vi "LV6_3.vi"() -> ()   [LabVIEW 2016]
uses:
  <vilib>/sound2/lvsound2.llb/Sampling Mode.ctl
  <vilib>/Utility/file.llb/Read From Spreadsheet File (DBL).vi
  <vilib>/imath/engines/lvmath2/RunTimeEngine/BuiltInFunctions/length/NIMS_length(GV).vi
  <instcachedir>/0/NIMS_length(GV)_08A3D13377FD4E4B96F5795FBF3698FA.lvgen/NIMS_length(GV)_08A3D13377FD4E4B96F5795FBF3698FA_000.vi
  <vilib>/imath/engines/lvmath2/RunTimeEngine/RangeToken/NIMS_Range.vi
  <instcachedir>/0/NIMS_Range_A7C094595B484CA7AF10685B02D808ED.lvgen/NIMS_Range_A7C094595B484CA7AF10685B02D808ED_001.vi
  <vilib>/imathl/engines/lvmath/Functions/Error Handling/Create Error.vi
  <vilib>/imath/engines/lvmath2/RunTimeEngine/BuiltInFunctions/randnormal/NIMS_randnormal(Str,I32).vi
  <vilib>/imath/engines/lvmath2/RunTimeEngine/BuiltInFunctions/randnormal/NIMS_randnormal(1,I32).vi
  <vilib>/imath/engines/lvmath2/RunTimeEngine/ArithmeticOperatorToken/NIMS_ArithmeticOperator_plus.vi
  <instcachedir>/0/NIMS_ArithmeticOperator_plus_0120E0498A0F4B4B9BDCAC2554767A4E.lvgen/NIMS_ArithmeticOperator_plus_0120E0498A0F4B4B9BDCAC2554767A4E_004.vi
  <vilib>/imath/engines/lvmath2/RunTimeEngine/ErrorHandling/NIMS_Error From Error Code.vi
  <vilib>/imath/engines/lvmath2/RunTimeEngine/BuiltInFunctions/poly/NIMS_GV=poly(GV).vi
  <instcachedir>/0/NIMS_GV=poly(GV)_A1C8B7C92C4F409DB664B03EC1C81090.lvgen/NIMS_GV=poly(GV)_A1C8B7C92C4F409DB664B03EC1C81090_000.vi
  <vilib>/imath/engines/lvmath2/RunTimeEngine/ErrorHandling/NIMS_Create Error From Enums.vi
  <vilib>/imath/engines/lvmath2/RunTimeEngine/BuiltInFunctions/residue/NIMS_residue_To Partial Fraction Expansion.vi
  <vilib>/imath/engines/lvmath2/RunTimeEngine/ArithmeticOperatorToken/NIMS_ArithmeticOperator_multmx.vi
  <instcachedir>/0/NIMS_ArithmeticOperator_multmx_4A56FE5C615140CE835D4DB5891BF065.lvgen/NIMS_ArithmeticOperator_multmx_4A56FE5C615140CE835D4DB5891BF065_006.vi
  <vilib>/imath/engines/lvmath2/RunTimeEngine/ArithmeticOperatorToken/NIMS_ArithmeticOperator_multmx(RV,M).vi
  <instcachedir>/0/NIMS_ArithmeticOperator_multmx(RV,M)_ECFE0528576D41C1AC80678C44A8AD28.lvgen/NIMS_ArithmeticOperator_multmx(RV,M)_ECFE0528576D41C1AC80678C44A8AD28_000.vi
  <vilib>/imath/engines/lvmath2/RunTimeEngine/BuiltInFunctions/fft/NIMS_fft(GM).vi
  <instcachedir>/0/NIMS_fft(GM)_7BD4D6367ED64442B25130C0D1EFC54B.lvgen/NIMS_fft(GM)_7BD4D6367ED64442B25130C0D1EFC54B_000.vi
  <vilib>/imath/engines/lvmath2/RunTimeEngine/BuiltInFunctions/fft/NIMS_fft(GV).vi
  <instcachedir>/0/NIMS_fft(GV)_4C6467FC22F84E4BA42517A07EF978B0.lvgen/NIMS_fft(GV)_4C6467FC22F84E4BA42517A07EF978B0_000.vi
  <vilib>/imath/engines/lvmath2/RunTimeEngine/ArithmeticOperatorToken/NIMS_ArithmeticOperator_times.vi
  <instcachedir>/0/NIMS_ArithmeticOperator_times_953B34F74CAC448FB707D816A29CC5F0.lvgen/NIMS_ArithmeticOperator_times_953B34F74CAC448FB707D816A29CC5F0_001.vi
  <vilib>/imath/engines/lvmath2/RunTimeEngine/BuiltInFunctions/ifft/NIMS_ifft(CM).vi
  <vilib>/imath/engines/lvmath2/RunTimeEngine/IndexRead/NIMS M(V).vi
  <instcachedir>/0/NIMS M(V)_948FAC22C1C943948B75DA6190348614.lvgen/NIMS M(V)_948FAC22C1C943948B75DA6190348614_004.vi
  <vilib>/imath/engines/lvmath2/RunTimeEngine/BuiltInFunctions/abs/NIMS_abs(signed).vi
  <instcachedir>/0/NIMS_abs(signed)_C4FCB8E6058B49B797C7C8D53CA5F6EC.lvgen/NIMS_abs(signed)_C4FCB8E6058B49B797C7C8D53CA5F6EC_003.vi
  <vilib>/imath/engines/lvmath2/RunTimeEngine/IndexRead/NIMS V(V).vi
  <instcachedir>/0/NIMS V(V)_298D9CB7BFEB42B8BC8D9C3C28AE8C70.lvgen/NIMS V(V)_298D9CB7BFEB42B8BC8D9C3C28AE8C70_000.vi
  <instcachedir>/0/NIMS_abs(signed)_C4FCB8E6058B49B797C7C8D53CA5F6EC.lvgen/NIMS_abs(signed)_C4FCB8E6058B49B797C7C8D53CA5F6EC_006.vi
  <vilib>/imath/engines/lvmath2/RunTimeEngine/NodeEndStatement/NIMS_NodeEndStatement_Output.vi
  <instcachedir>/0/NIMS_NodeEndStatement_Output_53EC0D466D134D7ABD903AC30B43404B.lvgen/NIMS_NodeEndStatement_Output_53EC0D466D134D7ABD903AC30B43404B_005.vi
  <instcachedir>/0/NIMS_NodeEndStatement_Output_53EC0D466D134D7ABD903AC30B43404B.lvgen/NIMS_NodeEndStatement_Output_53EC0D466D134D7ABD903AC30B43404B_002.vi
  <instcachedir>/0/NIMS_NodeEndStatement_Output_53EC0D466D134D7ABD903AC30B43404B.lvgen/NIMS_NodeEndStatement_Output_53EC0D466D134D7ABD903AC30B43404B_010.vi
  <vilib>/imath/engines/lvmath2/RunTimeEngine/ErrorHandling/NIMS_Finalize Error.vi
  <vilib>/imath/engines/lvmath2/RunTimeEngine/BuiltInFunctions/iir_butter/NIMS_[2o]_iir_butter(I32,V,Str).vi
  <vilib>/imath/engines/lvmath2/RunTimeEngine/BuiltInFunctions/findnz/NIMS_[1o]_findnz(GRowV).vi
  <instcachedir>/0/NIMS_[1o]_findnz(GRowV)_1AF74843B4874134ADE908C0A4A72F3C.lvgen/NIMS_[1o]_findnz(GRowV)_1AF74843B4874134ADE908C0A4A72F3C_000.vi
  <vilib>/imath/engines/lvmath2/RunTimeEngine/IndexReplace/NIMS V(V)=S.vi
  <instcachedir>/0/NIMS V(V)=S_4469BB7E0DD5440190F262393D16598E.lvgen/NIMS V(V)=S_4469BB7E0DD5440190F262393D16598E_002.vi
  <vilib>/imath/engines/lvmath2/RunTimeEngine/BuiltInFunctions/ifft/NIMS_ifft(CV).vi
  <instcachedir>/0/NIMS_ArithmeticOperator_times_953B34F74CAC448FB707D816A29CC5F0.lvgen/NIMS_ArithmeticOperator_times_953B34F74CAC448FB707D816A29CC5F0_000.vi
  <vilib>/imath/engines/lvmath2/RunTimeEngine/BuiltInFunctions/sum/NIMS_sum(GV).vi
  <instcachedir>/0/NIMS_sum(GV)_67F5EC36BC034E54A6BEC5B0673C00E5.lvgen/NIMS_sum(GV)_67F5EC36BC034E54A6BEC5B0673C00E5_000.vi
  <vilib>/sound2/lvsound2.llb/Sound Output Write (DBL Single).vi
panel:
  in  "stop":bool
  in  "Play filtered sound":bool
  in  "Play noisy sound":bool
  in  "Play original sound":bool
  in  "Noise level":dbl(knob)=0.2 scale=0.0..1.0
  out "Filtered signal (time domain)":cluster{"t":dbl[], "Y":dbl[]}(graph)
  out "Original signal (time domain)":cluster{"t":dbl[], "first row":dbl[]}(graph)
  out "Original signal (freq domain)":cluster{"F":dbl[], "FXI":dbl[]}(graph)
  out "Filtered signal (frequency domain)":cluster{"F":dbl[], "FZI":dbl[]}(graph)
  out "Nosiy signal (time domain)":cluster{"t":dbl[], "Y":dbl[]}(graph)
  out "Noisy signal (freq domain)":cluster{"F":dbl[], "FYI":dbl[]}[](graph)
  in  "Method":T1(tab)
  in  "order":i32(slide)=10 scale=2.0..10.0
  in  "minus real part of poles":dbl(slide)=10.0 scale=10.0..100.0
  in  "fundamental frequency (Hz)":dbl(slide)=491.0 scale=300.0..1000.0
  in  "order":i32(slide)=10 scale=2.0..10.0
  in  "cutoff frequency (Hz)":dbl(slide)=600.0 scale=1000.0..2500.0
  in  "Threshold":dbl(slide)=0.01 scale=0.0005..0.01
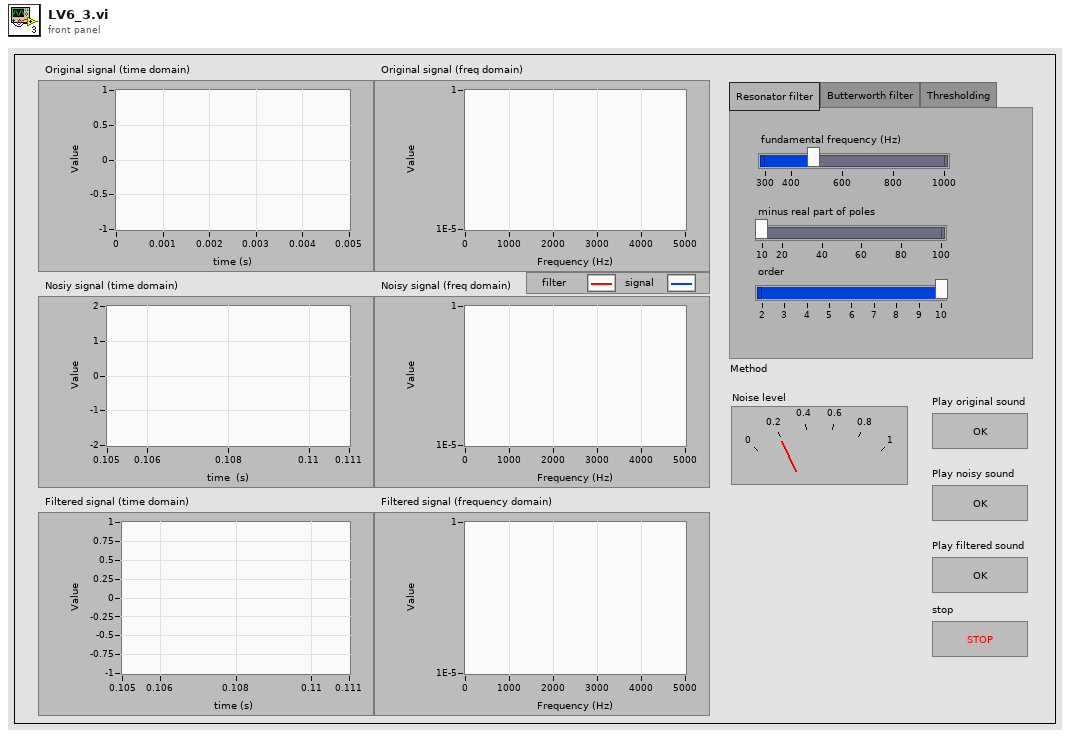
[diagram p1: front panel]
types:
  T1 = enum32{"Resonator filter", "Butterworth filter", "Thresholding"}
  T2 = typedef "Sampling Mode.ctl" = i32
  T3 = typedef "Sound Output Task ID.ctl" = u32
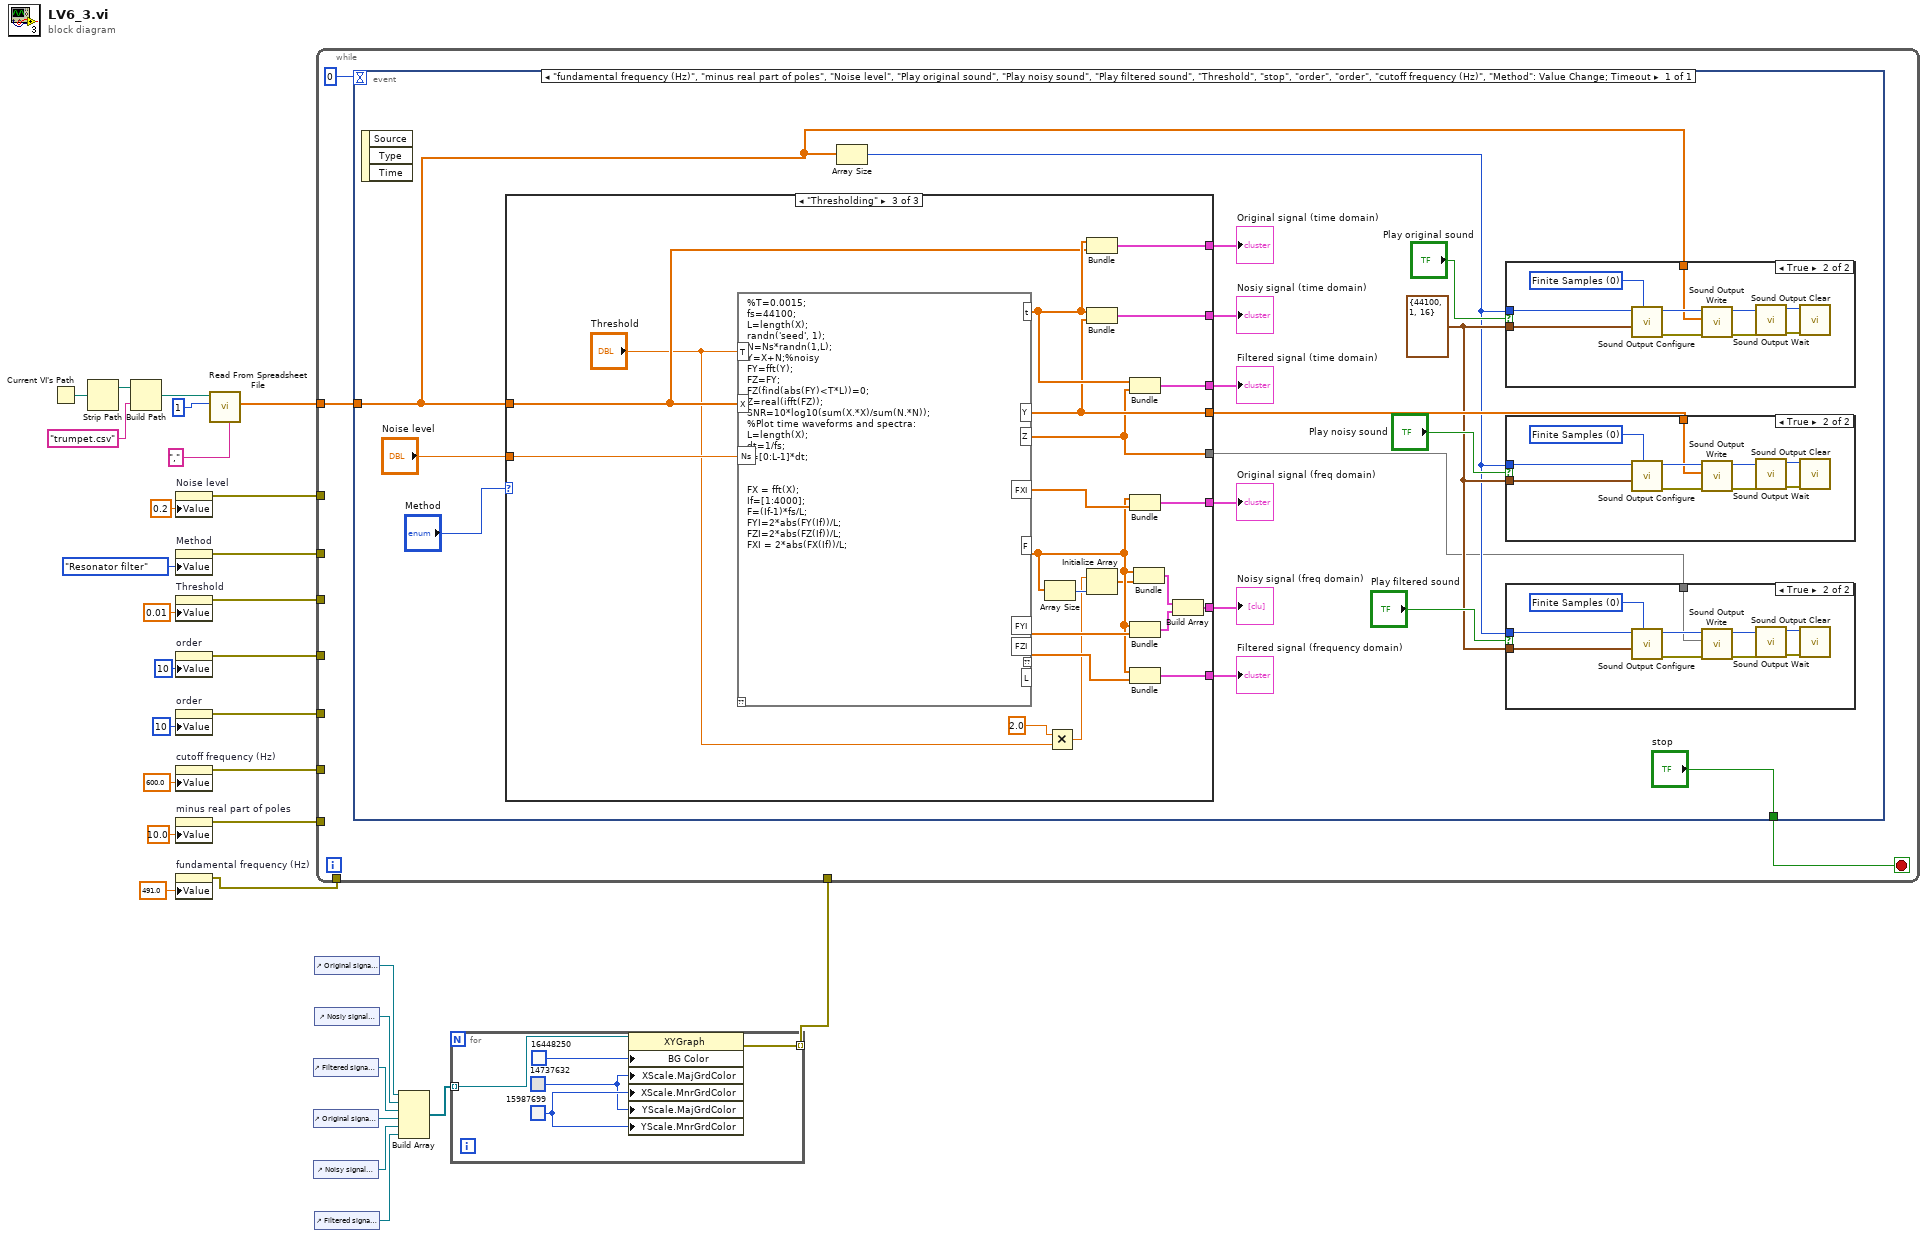
[diagram p0: block diagram]
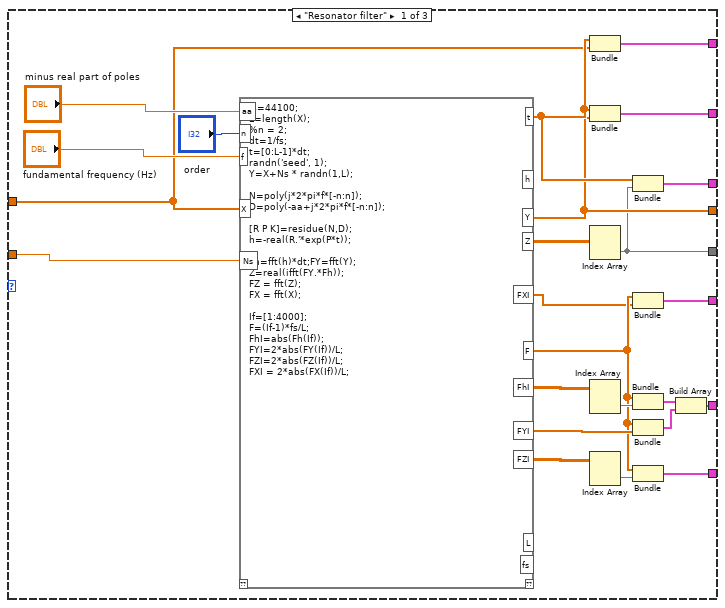
[diagram p5: hidden frame]
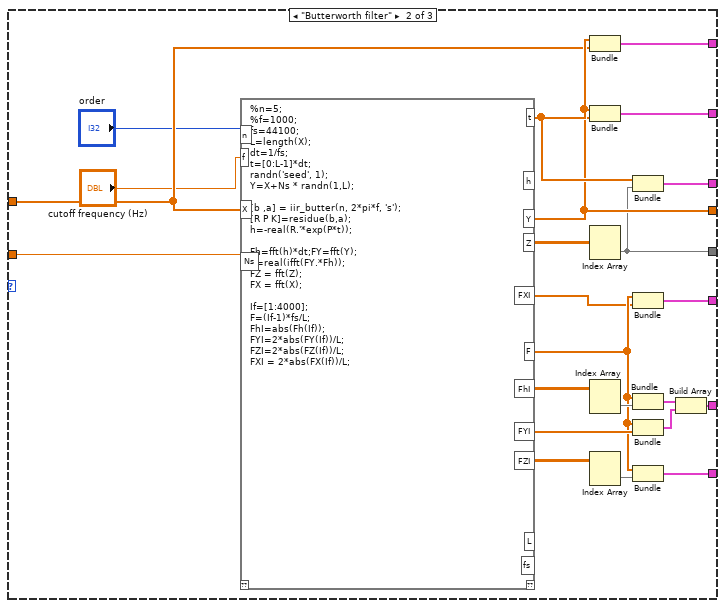
[diagram p6: hidden frame]
diagram:
  n1 = Current VI's Path() -> (path=w31:path)
  n2 = Strip Path(path=w31) -> (stripped path=w30:path)  [unwired: 1 out]
  n3 = Build Path(base path=w30, name or relative path="trumpet.csv") -> (appended path=w28:path)
  n4 = property on="Noise level" class="Knob (strict)"("Value"=0.2 ("Noise level")) -> (error out=w16:errorcluster)  [unwired: 2 in, 1 out]
  n5 = property on="Method" class="TabCtl (strict)"("Value"=T1."Resonator filter" ("Method")) -> (error out=w15:errorcluster)  [unwired: 2 in, 1 out]
  n6 = property on="Threshold" class="Slide (strict)"("Value"=0.01 ("Threshold")) -> (error out=w14:errorcluster)  [unwired: 2 in, 1 out]
  n7 = property on="order" class="Slide (strict)"("Value"=10 ("order")) -> (error out=w13:errorcluster)  [unwired: 2 in, 1 out]
  n8 = property on="order" class="Slide (strict)"("Value"=10 ("order")) -> (error out=w12:errorcluster)  [unwired: 2 in, 1 out]
  n9 = property on="cutoff frequency (Hz)" class="Slide (strict)"("Value"=600.0 ("cutoff frequency (Hz)")) -> (error out=w11:errorcluster)  [unwired: 2 in, 1 out]
  n10 = property on="minus real part of poles" class="Slide (strict)"("Value"=10.0 ("minus real part of poles")) -> (error out=w10:errorcluster)  [unwired: 2 in, 1 out]
  n11 = property on="fundamental frequency (Hz)" class="Slide (strict)"("Value"=491.0 ("fundamental frequency (Hz)")) -> (error out=w9:errorcluster)  [unwired: 2 in, 1 out]
  n12 = call-poly <vilib>:"Read From Spreadsheet File.vi"("delimiter (\\t)"="," ("delimiter (\\t)"), "number of rows (all:-1)"=1, "file path (dialog if empty)"=w28) -> ("first row"=w25:dbl[])  [unwired: 4 in, 4 out]
  n13 = control-ref of="Filtered signal (time domain)"() -> (w4:refnum<vi>)
  n14 = control-ref of="Original signal (freq domain)"() -> (w3:refnum<vi>)
  n15 = control-ref of="Noisy signal (freq domain)"() -> (w2:refnum<vi>)
  n16 = control-ref of="Original signal (time domain)"() -> (w6:refnum<vi>)
  n17 = control-ref of="Nosiy signal (time domain)"() -> (w5:refnum<vi>)
  n18 = control-ref of="Filtered signal (frequency domain)"() -> (w1:refnum<vi>)
  n19 = Build Array(w6, w5, w4, w3, w2, w1) -> (w8:refnum<vi>[])
  n20 = for {
    tunnel: w8 -> [w33] mode=indexing
    tunnel: [w32] -> w7 mode=indexing
    w35 = u32 15987699
    w34 = u32 14737632
    n21 = property class="XYGraph"(reference=w33, "BG Color"=u32 16448250, "XScale.MajGrdColor"=w34, "XScale.MnrGrdColor"=w35, "YScale.MajGrdColor"=w34, "YScale.MnrGrdColor"=w35) -> (error out=w32:errorcluster)  [unwired: 1 in, 1 out]
  }
  n22 = while {
    tunnel: w25 -> [w40]
    tunnel: w16 -> [_]
    tunnel: w15 -> [_]
    tunnel: w14 -> [_]
    tunnel: [w38] -> _
    tunnel: w13 -> [w38]
    tunnel: w12 -> [_]
    tunnel: w11 -> [_]
    tunnel: w10 -> [_]
    tunnel: w9 -> [_]
    tunnel: w7 -> [_]
    stop <- w39 stop-if-true
    n23 = event shown="[0] \"fundamental frequency (Hz)\", \"minus real part of poles\", \"Noise level\", \"Play original sound\", \"Play noisy sound\", \"Play filtered sound\", \"Threshold\", \"stop\", \"order\", \"order\", \"cutoff frequency (Hz)\", \"Method\": Value Change;  Timeout" {
      selector: _ -> [_]
      dyn-events: _ -> [_]
      timeout: 0 -> [_]
      tunnel: w40 -> [w48]
      tunnel: ["stop"] -> w39
      event "fundamental frequency (Hz)", "minus real part of poles", "Noise level", "Play original sound", "Play noisy sound", "Play filtered sound", "Threshold", "stop", "order", "order", "cutoff frequency (Hz)", "Method": Value Change; Timeout {
        w44 = cluster{"fs":i32, i32, i32} {"fs"=44100, 1, 16}
        n24 = event-data() -> ()  [unwired: 1 in, 3 out]
        n25 = case shown="\"Thresholding\"" "Method" {
          tunnel: [w103 w607 w1072] -> w57
          tunnel: [w99 w603 w1071] -> w56
          tunnel: [w97 w601 w1070] -> w55
          tunnel: [w96 w600 w1069] -> w54
          tunnel: w48 -> [w94 w598 w1067]
          tunnel: [w93 w597 w1066] -> w53
          tunnel: [w92 w596 w1065] -> w52
          tunnel: "Noise level" -> [w91 w591 w1064]
          tunnel: [w90 w595 w1063] -> w46
          tunnel: [w89 w594 w1060] -> w42
          frame "Resonator filter" {
            n26 = mathscript code="fs=44100;\nL=length(X);\n%n = 2;\ndt=1/fs;\nt=[0:L-1]*dt;\nrandn('seed', 1);\nY=X+Ns * randn(1,L);\n\nN=poly(j*2*pi*f*[-n:n]);\nD=poly(-aa+j*2*pi*f*[-n:n]);\n\n[R P K]=residue(N,D);\nh=-real(R.'*exp(P*t));\n\nFh=fft(h)*dt;FY=fft(Y);\nZ=real(ifft(FY.*Fh));\nFZ = fft(Z);\nFX = fft(X);\n\nIf=[1:4000];\nF=(If-1)*fs/L;\nFhI=abs(Fh(If));\nFYI=2*abs(FY(If))/L;\nFZI=2*abs(FZ(If))/L;\nFXI = 2*abs(FX(If))/L;"("X"=w94, "aa"="minus real part of poles", "n"="order", "f"="fundamental frequency (Hz)", "Ns"=w91) -> ("Z"=w102:dbl[][], "Y"=w90:dbl[], "F"=w98:dbl[], "FhI"=w108:dbl[][], "FYI"=w106:dbl[], "t"=w95:dbl[], "FZI"=w101:dbl[][], "FXI"=w88:dbl[])  [unwired: 1 in, 4 out]
            n27 = Bundle("t"=w95, "first row"=w94) -> (w93:cluster{"t":dbl[], "first row":dbl[]})  [unwired: 1 in]
            n28 = Bundle("t"=w95, "Y"=w90) -> (w96:cluster{"t":dbl[], "Y":dbl[]})  [unwired: 1 in]
            n29 = Index Array(array=w102) -> (element=w89:dbl[])  [unwired: 2 in]
            n30 = Index Array(array=w108) -> (element=w107:dbl[])  [unwired: 2 in]
            n31 = Index Array(array=w101) -> (element=w100:dbl[])  [unwired: 2 in]
            n32 = Bundle("t"=w95, "Z"=w89) -> (w92:cluster{"t":dbl[], "Z":dbl[]})  [unwired: 1 in]
            n33 = Bundle("F"=w98, "FXI"=w88) -> (w97:cluster{"F":dbl[], "FXI":dbl[]})  [unwired: 1 in]
            n34 = Bundle("F"=w98, "FhI"=w107) -> (w105:cluster{"F":dbl[], "FhI":dbl[]})  [unwired: 1 in]
            n35 = Bundle("F"=w98, "FYI"=w106) -> (w104:cluster{"F":dbl[], "FYI":dbl[]})  [unwired: 1 in]
            n36 = Bundle("F"=w98, "FZI"=w100) -> (w99:cluster{"F":dbl[], "FZI":dbl[]})  [unwired: 1 in]
            n37 = Build Array(w105, w104) -> (w103:cluster{"F":dbl[], "FYI":dbl[]}[])
          }
          frame "Butterworth filter" {
            n38 = mathscript code="%n=5;\n%f=1000;\nfs=44100;\nL=length(X);\ndt=1/fs;\nt=[0:L-1]*dt;\nrandn('seed', 1);\nY=X+Ns * randn(1,L);\n\n[b ,a] = iir_butter(n, 2*pi*f, 's');\n[R P K]=residue(b,a);\nh=-real(R.'*exp(P*t));\n\nFh=fft(h)*dt;FY=fft(Y);\nZ=real(ifft(FY.*Fh));\nFZ = fft(Z);\nFX = fft(X);\n\nIf=[1:4000];\nF=(If-1)*fs/L;\nFhI=abs(Fh(If));\nFYI=2*abs(FY(If))/L;\nFZI=2*abs(FZ(If))/L;\nFXI = 2*abs(FX(If))/L;"("X"=w598, "n"="order", "f"="cutoff frequency (Hz)", "Ns"=w591) -> ("Z"=w606:dbl[][], "Y"=w595:dbl[], "F"=w602:dbl[], "FhI"=w612:dbl[][], "FYI"=w610:dbl[], "t"=w599:dbl[], "FZI"=w605:dbl[][], "FXI"=w590:dbl[])  [unwired: 1 in, 4 out]
            n39 = Bundle("t"=w599, "first row"=w598) -> (w597:cluster{"t":dbl[], "first row":dbl[]})  [unwired: 1 in]
            n40 = Bundle("t"=w599, "Y"=w595) -> (w600:cluster{"t":dbl[], "Y":dbl[]})  [unwired: 1 in]
            n41 = Index Array(array=w606) -> (element=w594:dbl[])  [unwired: 2 in]
            n42 = Index Array(array=w612) -> (element=w611:dbl[])  [unwired: 2 in]
            n43 = Index Array(array=w605) -> (element=w604:dbl[])  [unwired: 2 in]
            n44 = Bundle("t"=w599, "Z"=w594) -> (w596:cluster{"t":dbl[], "Z":dbl[]})  [unwired: 1 in]
            n45 = Bundle("F"=w602, "FXI"=w590) -> (w601:cluster{"F":dbl[], "FXI":dbl[]})  [unwired: 1 in]
            n46 = Bundle("F"=w602, "FhI"=w611) -> (w609:cluster{"F":dbl[], "FhI":dbl[]})  [unwired: 1 in]
            n47 = Bundle("F"=w602, "FYI"=w610) -> (w608:cluster{"F":dbl[], "FYI":dbl[]})  [unwired: 1 in]
            n48 = Bundle("F"=w602, "FZI"=w604) -> (w603:cluster{"F":dbl[], "FZI":dbl[]})  [unwired: 1 in]
            n49 = Build Array(w609, w608) -> (w607:cluster{"F":dbl[], "FYI":dbl[]}[])
          }
          frame "Thresholding" {
            n50 = mathscript code="%T=0.0015;\nfs=44100;\nL=length(X);\nrandn('seed', 1);\nN=Ns*randn(1,L);\nY=X+N;%noisy\nFY=fft(Y);\nFZ=FY;\nFZ(find(abs(FY)<T*L))=0;\nZ=real(ifft(FZ));\nSNR=10*log10(sum(X.*X)/sum(N.*N));\n%Plot time waveforms and spectra:\nL=length(X);\ndt=1/fs;\nt=[0:L-1]*dt;\n\n\nFX = fft(X);\nIf=[1:4000];\nF=(If-1)*fs/L;\nFYI=2*abs(FY(If))/L;\nFZI=2*abs(FZ(If))/L;\nFXI = 2*abs(FX(If))/L;"("X"=w1067, "T"="Threshold", "Ns"=w1064) -> ("Z"=w1060:dbl[], "Y"=w1063:dbl[], "F"=w1057:dbl[], "FYI"=w1073:dbl[], "t"=w1068:dbl[], "FZI"=w1061:dbl[], "FXI"=w1062:dbl[])  [unwired: 1 in, 2 out]
            n51 = Array Size(array=w1057) -> (size(s)=w1055:i32)
            n52 = Multiply(x=2.0 ("y"), y="Threshold") -> (x*y=w1054:dbl)
            n53 = Bundle("t"=w1068, "first row"=w1067) -> (w1066:cluster{"t":dbl[], "first row":dbl[]})  [unwired: 1 in]
            n54 = Bundle("t"=w1068, "Y"=w1063) -> (w1069:cluster{"t":dbl[], "Y":dbl[]})  [unwired: 1 in]
            n55 = Initialize Array(w1054, w1055) -> (w1056:dbl[])
            n56 = Bundle("t"=w1068, "Z"=w1060) -> (w1065:cluster{"t":dbl[], "Z":dbl[]})  [unwired: 1 in]
            n57 = Bundle("F"=w1057, "FXI"=w1062) -> (w1070:cluster{"F":dbl[], "FXI":dbl[]})  [unwired: 1 in]
            n58 = Bundle("F"=w1057, "FYI"=w1073) -> (w1059:cluster{"F":dbl[], "FYI":dbl[]})  [unwired: 1 in]
            n59 = Bundle("F"=w1057, "FZI"=w1061) -> (w1071:cluster{"F":dbl[], "FZI":dbl[]})  [unwired: 1 in]
            n60 = Bundle("F"=w1057, w1056) -> (w1058:cluster{"F":dbl[], dbl[]})  [unwired: 1 in]
            n61 = Build Array(w1058, w1059) -> (w1072:cluster{"F":dbl[], "FYI":dbl[]}[])
          }
        }
        "Noisy signal (freq domain)" <- w57
        "Nosiy signal (time domain)" <- w54
        "Filtered signal (frequency domain)" <- w56
        "Original signal (freq domain)" <- w55
        "Original signal (time domain)" <- w53
        "Filtered signal (time domain)" <- w52
        n62 = Array Size(array=w48) -> (size(s)=w43:i32)
        n63 = case shown="True" "Play original sound" {
          tunnel: w44 -> [_ w81]
          tunnel: w43 -> [_ w79]
          tunnel: w48 -> [_ w78]
          frame False {
          }
          frame True {
            w80 = T2 0 items=["Finite Samples", "Continuous Samples"] ("sample mode")
            n64 = call <vilib>:"Sound Output Configure.vi"("number of samples/ch"=w79, "sample mode"=w80, "sound format"=w81) -> ("error out"=w82:errorcluster, "task ID"=w87:T3)  [unwired: 7 in]
            n65 = call-poly <vilib>:"Sound Output Write.vi"("error in (no error)"=w82, "data"=w78, "task ID"=w87) -> ("error out"=w83:errorcluster, "task ID out"=w84:T3)  [unwired: 7 in]
            n66 = call <vilib>:"Sound Output Wait.vi"("error in (no error)"=w83, "task ID"=w84) -> ("error out"=w86:errorcluster, "task ID out"=w85:T3)  [unwired: 8 in]
            n67 = call <vilib>:"Sound Output Clear.vi"("error in (no error)"=w86, "task ID"=w85) -> ()  [unwired: 9 in, 1 out]
          }
        }
        n68 = case shown="True" "Play noisy sound" {
          tunnel: w44 -> [_ w71]
          tunnel: w43 -> [_ w69]
          tunnel: w46 -> [_ w68]
          frame False {
          }
          frame True {
            w70 = T2 0 items=["Finite Samples", "Continuous Samples"] ("sample mode")
            n69 = call <vilib>:"Sound Output Configure.vi"("number of samples/ch"=w69, "sample mode"=w70, "sound format"=w71) -> ("error out"=w72:errorcluster, "task ID"=w77:T3)  [unwired: 7 in]
            n70 = call-poly <vilib>:"Sound Output Write.vi"("error in (no error)"=w72, "data"=w68, "task ID"=w77) -> ("error out"=w73:errorcluster, "task ID out"=w74:T3)  [unwired: 7 in]
            n71 = call <vilib>:"Sound Output Wait.vi"("error in (no error)"=w73, "task ID"=w74) -> ("error out"=w76:errorcluster, "task ID out"=w75:T3)  [unwired: 8 in]
            n72 = call <vilib>:"Sound Output Clear.vi"("error in (no error)"=w76, "task ID"=w75) -> ()  [unwired: 9 in, 1 out]
          }
        }
        n73 = case shown="True" "Play filtered sound" {
          tunnel: w44 -> [_ w61]
          tunnel: w43 -> [_ w59]
          tunnel: w42 -> [_ w58]
          frame False {
          }
          frame True {
            w60 = T2 0 items=["Finite Samples", "Continuous Samples"] ("sample mode")
            n74 = call <vilib>:"Sound Output Configure.vi"("number of samples/ch"=w59, "sample mode"=w60, "sound format"=w61) -> ("error out"=w62:errorcluster, "task ID"=w67:T3)  [unwired: 7 in]
            n75 = call-poly <vilib>:"Sound Output Write.vi"("error in (no error)"=w62, "data"=w58, "task ID"=w67) -> ("error out"=w63:errorcluster, "task ID out"=w64:T3)  [unwired: 7 in]
            n76 = call <vilib>:"Sound Output Wait.vi"("error in (no error)"=w63, "task ID"=w64) -> ("error out"=w66:errorcluster, "task ID out"=w65:T3)  [unwired: 8 in]
            n77 = call <vilib>:"Sound Output Clear.vi"("error in (no error)"=w66, "task ID"=w65) -> ()  [unwired: 9 in, 1 out]
          }
        }
      }
    }
  }
